vi "communication.vi"() -> ()   [LabVIEW 2011]
uses:
  <vilib>/Instr/_visa.llb/VISA Configure Serial Port (Instr).vi
panel:
  out "standard output":string
  in  "file path (use dialog)":path=path "C:/tyrmt/data.csv.txt"
  out "error out":errorcluster
  in  "error in (no error)":errorcluster
  out "State buffer":string
  in  "State":bool
  in  "Reset":bool
  in  "Data":bool
  in  "VISA resource name":refnum<visa-resource-name>="COM4"
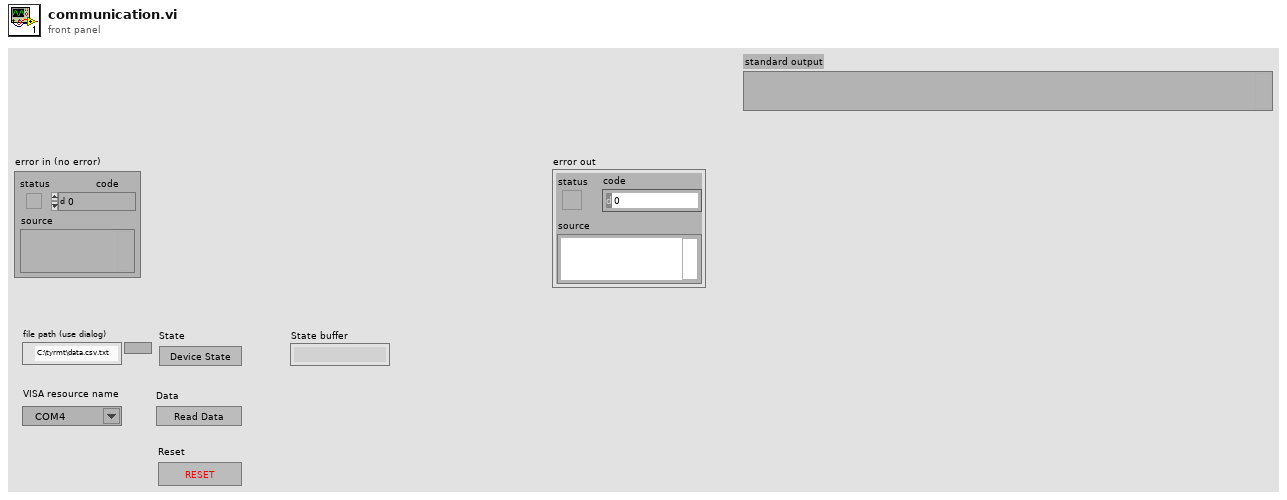
[diagram p1: front panel]
types:
  T1 = enum16{"open", "replace", "create", "open or create", "replace or create", "replace or create with confirmation"}
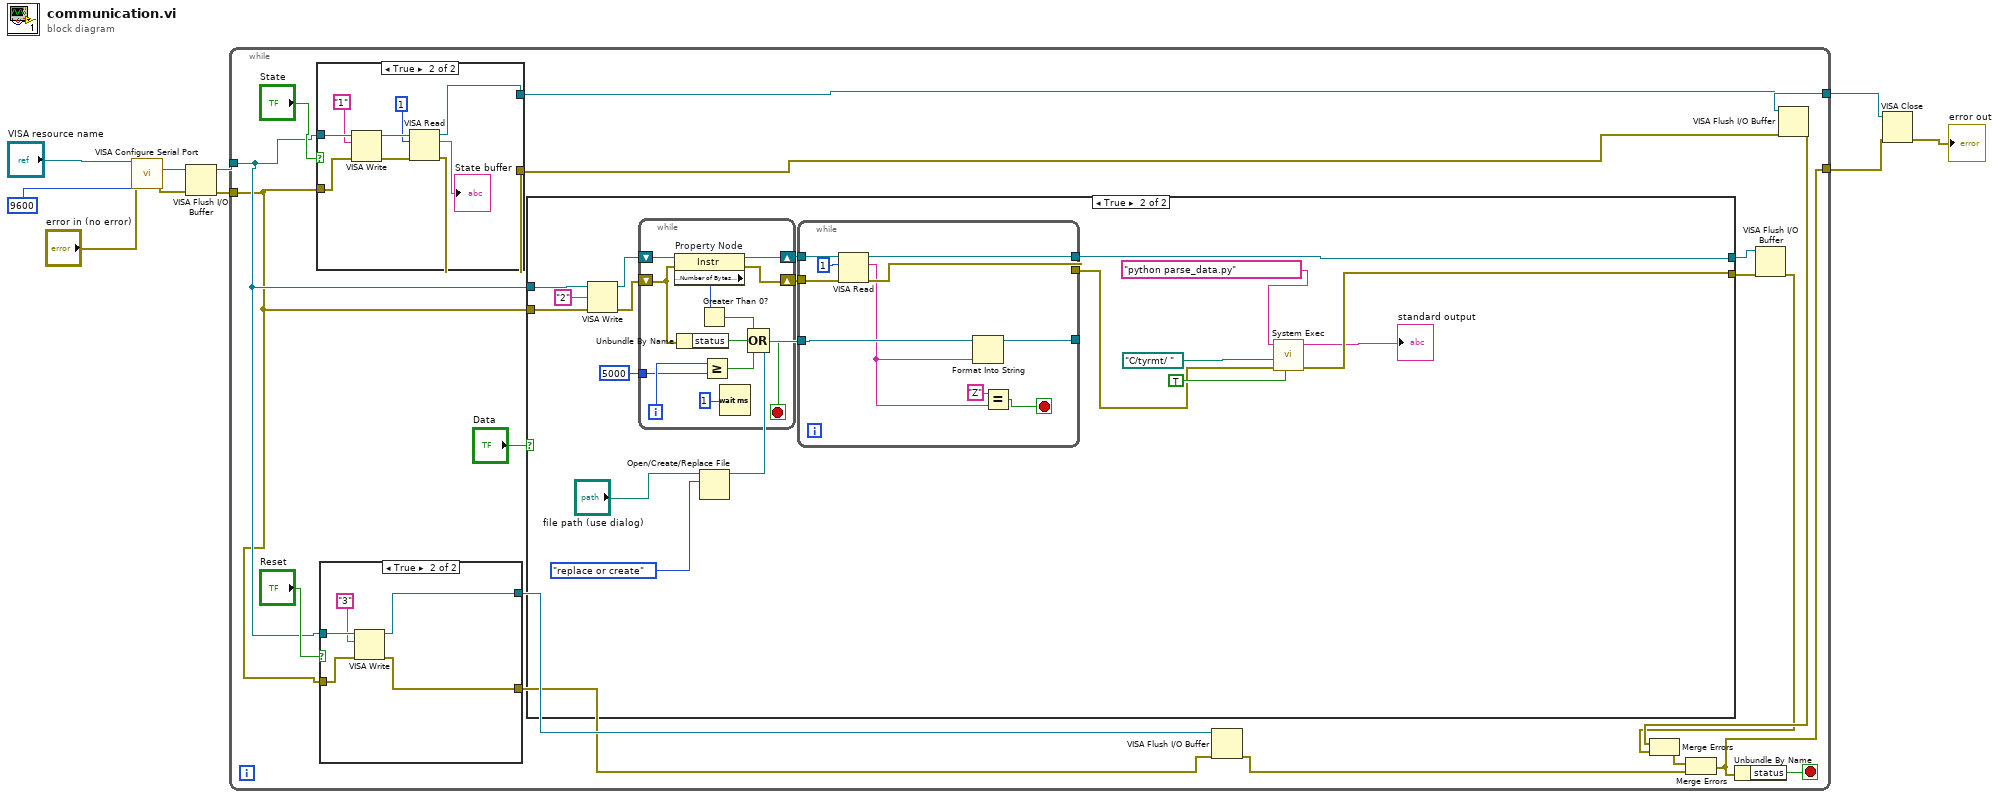
[diagram p0: block diagram]
diagram:
  n1 = call-poly "VISA Configure Serial Port"("VISA resource name"="VISA resource name", "baud rate (9600)"=9600, "error in (no error)"="error in (no error)") -> ("VISA resource name out"=w9:refnum<visa-resource-name>, "error out"=w8:errorcluster)  [unwired: 11 in]
  n2 = VISA Flush I/O Buffer(VISA resource name=w9, error in (no error)=w8) -> (VISA resource name out=w6:refnum<visa-resource-name>, error out=w5:errorcluster)  [unwired: 1 in]
  n3 = while {
    tunnel: w6 -> [w24]
    tunnel: w5 -> [w23]
    tunnel: [w13] -> w4
    tunnel: [w22] -> w3
    stop <- w26 stop-if-true
    n4 = case shown="True" "State" {
      tunnel: w24 -> [w79 w88]
      tunnel: w23 -> [w78 w87]
      tunnel: [w79 w82] -> w12
      tunnel: [w78 w81] -> w17
      frame False {
      }
      frame True {
        n5 = VISA Write(VISA resource name=w88, write buffer="1", error in (no error)=w87) -> (VISA resource name out=w84:refnum<visa-resource-name>, error out=w85:errorcluster)  [unwired: 1 out]
        n6 = VISA Read(VISA resource name=w84, byte count=1, error in (no error)=w85) -> (VISA resource name out=w82:refnum<visa-resource-name>, read buffer=→"State buffer":string, error out=w81:errorcluster)  [unwired: 1 out]
      }
    }
    n7 = case shown="True" "Reset" {
      tunnel: w24 -> [w72 w77]
      tunnel: w23 -> [w71 w76]
      tunnel: [w72 w74] -> w21
      tunnel: [w71 w73] -> w20
      frame False {
      }
      frame True {
        n8 = VISA Write(VISA resource name=w77, write buffer="3", error in (no error)=w76) -> (VISA resource name out=w74:refnum<visa-resource-name>, error out=w73:errorcluster)  [unwired: 1 out]
      }
    }
    n9 = case shown="True" "Data" {
      tunnel: w24 -> [w30 w48]
      tunnel: w23 -> [w29 w47]
      tunnel: [w30 w40] -> w18
      tunnel: [w29 w33] -> w16
      frame False {
      }
      frame True {
        n10 = VISA Write(VISA resource name=w48, write buffer="2", error in (no error)=w47) -> (VISA resource name out=w45:refnum<visa-resource-name>, error out=w44:errorcluster)  [unwired: 1 out]
        n11 = while {
          shift-right: [w69] -> w42
          shift-left: w45 -> [w70]
          shift-right: [w68] -> w41
          shift-left: w44 -> [w66]
          tunnel: 5000 ("Timeout (mS)") -> [w64]
          i -> [w65]
          stop <- w60 stop-if-true
          n12 = property on="Property Node" class="Instr"(reference=w70, error in=w66) -> (reference out=w69:refnum<visa-resource-name>, error out=w68:errorcluster, "Serial Settings:Number of Bytes at Serial Port"=w67:u32)
          n13 = Unbundle By Name(w66) -> ("status"=w62:bool)
          n14 = Greater Than 0?(x=w67) -> (x > 0?=w63:bool)
          n15 = Greater Or Equal?(x=w65, y=w64) -> (x >= y?=w61:bool)
          n16 = Wait (ms)(milliseconds to wait=u32 1) -> ()  [unwired: 1 out]
          n17 = Compound Arithmetic op=OR(w63, w62, w61) -> (w60:bool)
        }
        n18 = Open/Create/Replace File(file path (use dialog)="file path (use dialog)", operation (0:open)=T1."replace or create") -> (refnum out=w38:refnum<file>)  [unwired: 4 in, 2 out]
        n19 = while {
          tunnel: w42 -> [w57]
          tunnel: w41 -> [w58]
          tunnel: [w54] -> w40
          tunnel: [w53] -> w34
          tunnel: w38 -> [w51]
          tunnel: [w50] -> _
          stop <- w56 stop-if-true
          n20 = VISA Read(VISA resource name=w57, byte count=u32 1, error in (no error)=w58) -> (VISA resource name out=w54:refnum<visa-resource-name>, read buffer=w49:string, error out=w53:errorcluster)  [unwired: 1 out]
          n21 = Format Into String(initial string=w51, w49) -> (resulting string=w50:refnum<file>)  [unwired: 2 in, 1 out]
          n22 = Equal?(x="Z", y=w49) -> (x = y?=w56:bool)
        }
        n23 = call <vilib>:"System Exec.vi"("run minimized? (F)"=TRUE, "error in (no error)"=w34, "working directory"=path "C:/tyrmt/ ", "command line"="python parse_data.py") -> ("error out"=w33:errorcluster, "standard output"=→"standard output":string)  [unwired: 4 in, 2 out]
      }
    }
    n24 = VISA Flush I/O Buffer(VISA resource name=w21, error in (no error)=w20) -> (error out=w19:errorcluster)  [unwired: 1 in, 1 out]
    n25 = VISA Flush I/O Buffer(VISA resource name=w18, error in (no error)=w16) -> (error out=w11:errorcluster)  [unwired: 1 in, 1 out]
    n26 = VISA Flush I/O Buffer(VISA resource name=w12, error in (no error)=w17) -> (VISA resource name out=w13:refnum<visa-resource-name>, error out=w14:errorcluster)  [unwired: 1 in]
    n27 = Merge Errors(w14, w11) -> (w15:errorcluster)
    n28 = Merge Errors(w15, w19) -> (w22:errorcluster)
    n29 = Unbundle By Name(w22) -> ("status"=w26:bool)
  }
  n30 = VISA Close(VISA resource name=w4, error in (no error)=w3) -> (error out=→"error out":errorcluster)
